vi "PowerDmm.vi"() -> ()   [LabVIEW 2015]
uses:
  <vilib>/RAFA Solutions/Rainbow Flat UI Controls Kit (Light)/Boolean/Radio Button.ctl
  <vilib>/RAFA Solutions/Rainbow Flat UI Controls Kit (Light)/Numeric/Numeric Indicator.ctl
  <vilib>/RAFA Solutions/Rainbow Flat UI Controls Kit (Light)/Numeric/Dial Simple.ctl
  <vilib>/RAFA Solutions/Rainbow Flat UI Controls Kit (Light)/Boolean/Slide Switch Round.ctl
  <vilib>/VirtualBench/_DMM Configure Measurement4.vi
  <vilib>/VirtualBench/_PS Configure Voltage Output0.vi
  <vilib>/VirtualBench/VirtualBench.lvlib
  <vilib>/RAFA Solutions/Rainbow Flat UI Controls Kit (Light)/Rainbow Light.lvlib
panel:
  in  "Auto Range Terminal":i32(ring) items=["Low", "High"]
  in  "Power Channel":tag="VB8012-3060439/ps/+6V"
  out "Analog Data":cluster{dbl[], dbl[]}(graph)
  in  "Voltage Level (V)":dbl(slide)=2.0 caption="Current Limit (no change)" scale=0.0..25.0
  in  "Current Limit (A)":dbl(slide)=0.1 caption="Current Limit (no change)" scale=0.0..1.0
  in  "milliseconds to wait":u32=30
  in  "deltaV":dbl=0.2 format="%#_13g"
  in  "Vlow":dbl format="%#_13g"
  in  "Vhigh":dbl=6.0 format="%#_13g"
  in  "Voltage Ramp":T1
  out "Actual Voltage Level":T2 scale=0.0..2.0
  out "Actual Current":T2 scale=0.0..2.0
  out "Calculated Resistance":T3
  out "DMM Reading":dbl(knob)=20.92102921572232 scale=0.0..25.0
  out "DMM Reading (Waveform)":dbl(graph)
  in  "Auto Range":T4=TRUE caption="Auto Range (no change)"
  in  "Function":i32(ring) caption="Function (no change)" items=["DC Volts", "AC Volts", "DC Current", "AC Current", "Resistance", "Diode"]
  in  "stop":bool
  in  "Enable Outputs":T4
  in  "Power Channel":tag="ps/+6V" caption="Channel"
  in  "Device Name":tag="VB8012-3060439"
  # "Power Supply Configuration"
  # "Power Supply Output"
  # "Digital Multimeter"
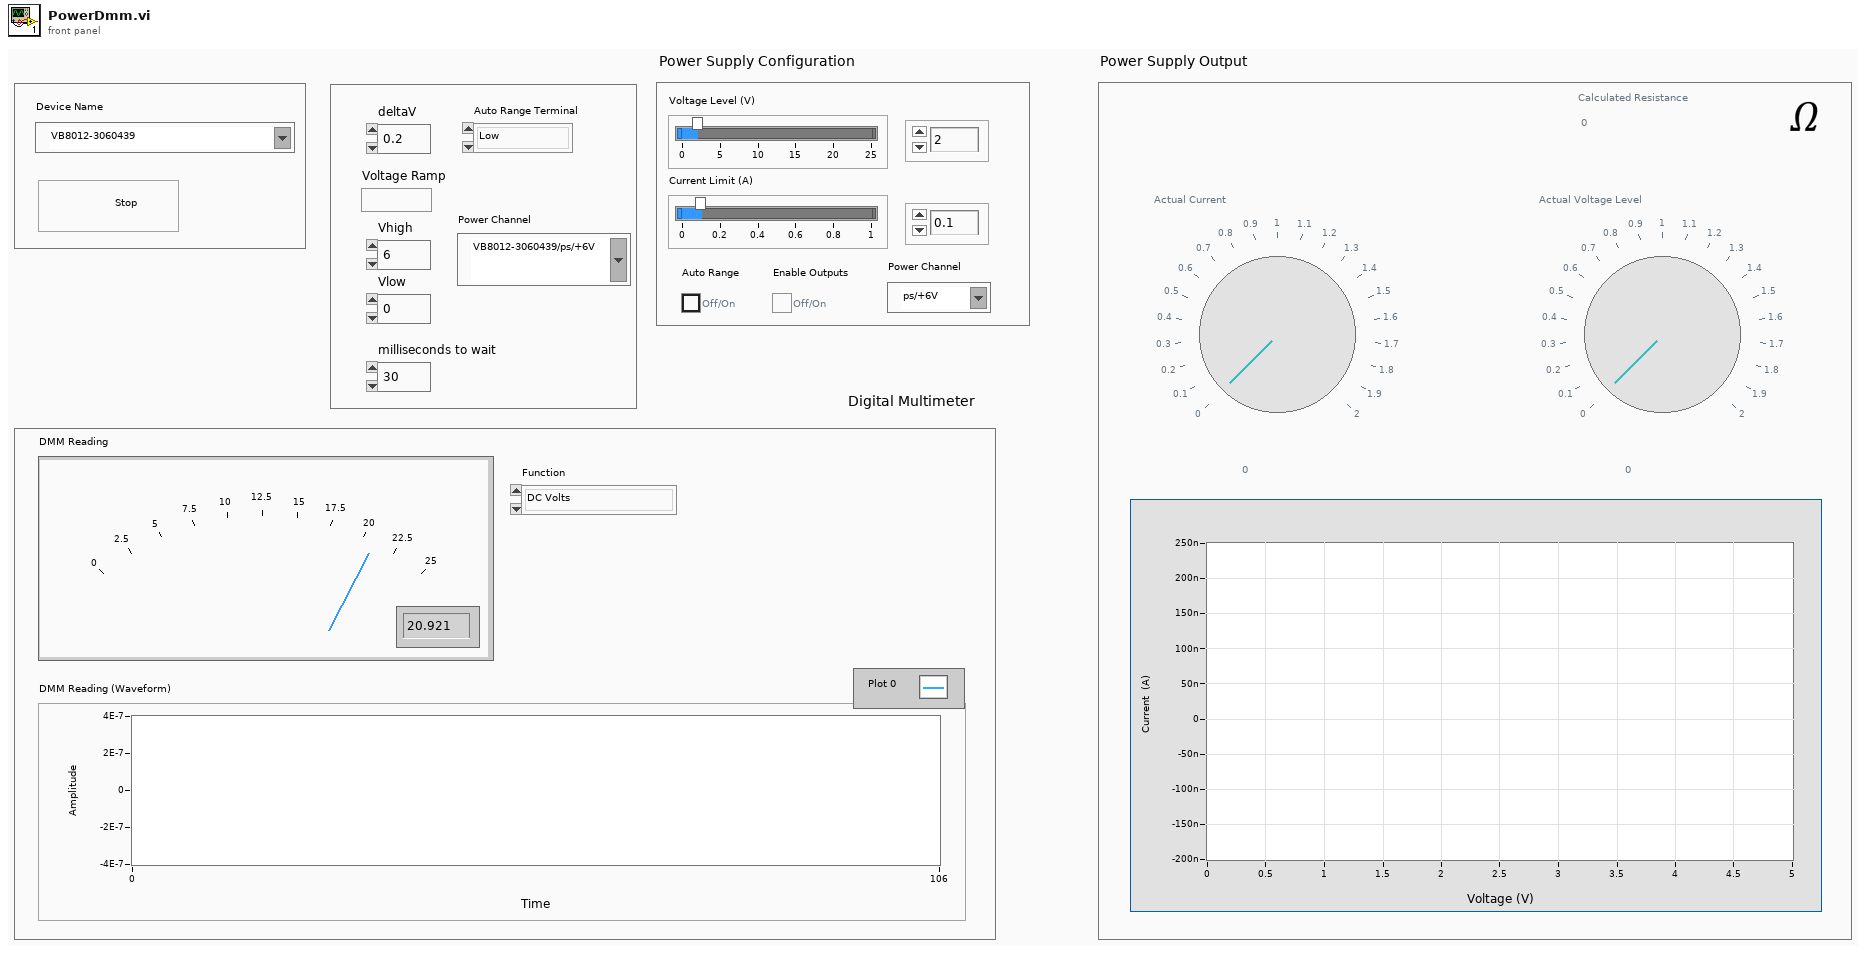
[diagram p1: front panel]
types:
  T1 = typedef "Rainbow Light.lvlib/Slide Switch Round.ctl" = bool
  T2 = typedef "Rainbow Light.lvlib/Dial Simple.ctl" = dbl
  T3 = typedef "Rainbow Light.lvlib/Numeric Indicator.ctl" = dbl
  T4 = typedef "Rainbow Light.lvlib/Radio Button.ctl" = bool
  T5 = cluster{"milliseconds to wait":u32, "deltaV":dbl, "Vhigh":dbl, "Vlow":dbl}
  T6 = cluster{"Instrument Handle Out":refnum<k21>, "Instrument Handle Out":refnum<k21>}
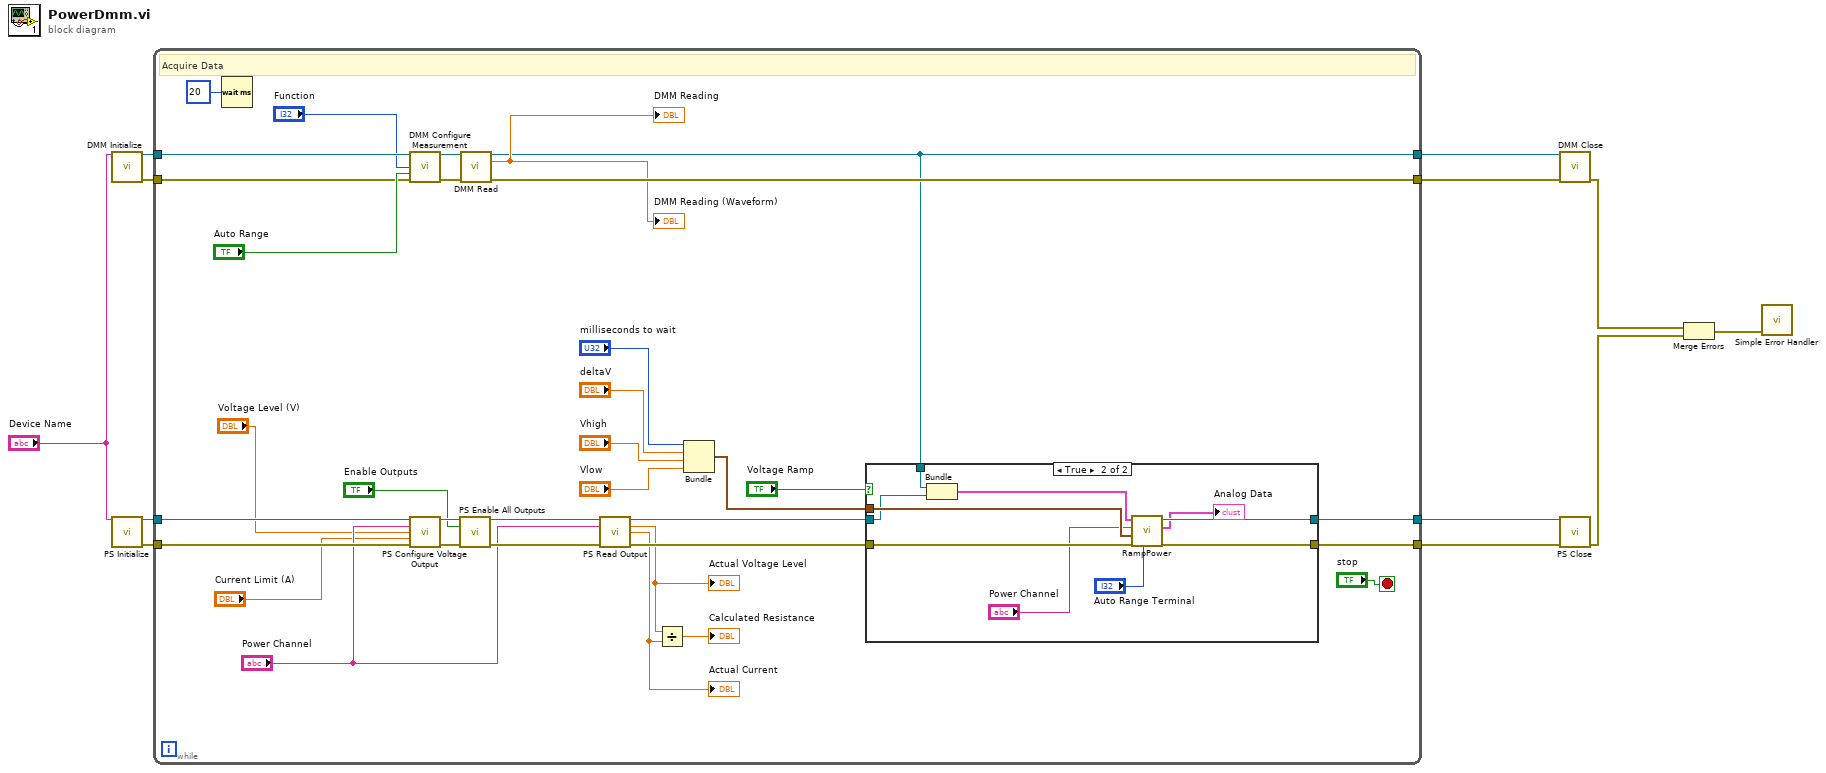
[diagram p0: block diagram]
diagram:
  n1 = call <vilib>:"DMM Initialize.vi"("Device Name"="Device Name") -> ("Instrument Handle Out"=w8:refnum<k21>, "Error Out"=w7:errorcluster)  [unwired: 13 in]
  n2 = call <vilib>:"PS Initialize.vi"("Device Name"="Device Name") -> ("Instrument Handle Out"=w12:refnum<k21>, "Error Out"=w11:errorcluster)  [unwired: 13 in]
  n3 = while {
    tunnel: w12 -> [w46]
    tunnel: w11 -> [w45]
    tunnel: [w27] -> w10
    tunnel: w8 -> [w39]
    tunnel: w7 -> [w35]
    tunnel: [w34] -> w6
    tunnel: [w26] -> w5
    tunnel: [w13] -> w4
    stop <- "stop" stop-if-true
    # "Acquire Data"
    n4 = Wait (ms)(milliseconds to wait=u32 20) -> ()  [unwired: 1 out]
    n5 = call-poly <vilib>:"DMM Configure Measurement.vi"("Instrument Handle In"=w39, "Function"="Function", "Auto Range"="Auto Range", "Error In"=w35) -> ("Instrument Handle Out"=w37:refnum<k21>, "Error Out"=w36:errorcluster)  [unwired: 10 in]
    n6 = call-poly <vilib>:"PS Configure Voltage Output.vi"("Instrument Handle In"=w46, "Channel"="Power Channel", "Voltage Level"="Voltage Level (V)", "Current Limit"="Current Limit (A)", "Error In"=w45) -> ("Instrument Handle Out"=w44:refnum<k21>, "Error Out"=w43:errorcluster)  [unwired: 9 in]
    n7 = call <vilib>:"PS Enable All Outputs.vi"("Instrument Handle In"=w44, "Enable Outputs"="Enable Outputs", "Error In"=w43) -> ("Instrument Handle Out"=w33:refnum<k21>, "Error Out"=w32:errorcluster)  [unwired: 11 in]
    n8 = call <vilib>:"DMM Read.vi"("Instrument Handle In"=w37, "Error In"=w36) -> ("Instrument Handle Out"=w13:refnum<k21>, "Measurement"=→"DMM Reading (Waveform)" →"DMM Reading":dbl, "Error Out"=w34:errorcluster)  [unwired: 11 in]
    n9 = call <vilib>:"PS Read Output.vi"("Instrument Handle In"=w33, "Channel"="Power Channel", "Error In"=w32) -> ("Instrument Handle Out"=w29:refnum<k21>, "Actual Voltage Level"=w17:dbl, "Actual Current Level"=w20:dbl, "Error Out"=w28:errorcluster)  [unwired: 8 in, 1 out]
    "Actual Current" <- w20
    "Actual Voltage Level" <- w17
    n10 = Divide(x=w17, y=w20) -> (x/y=→"Calculated Resistance":dbl)
    n11 = Bundle("milliseconds to wait"="milliseconds to wait", "deltaV"="deltaV", "Vhigh"="Vhigh", "Vlow"="Vlow") -> (w25:T5)  [unwired: 1 in]
    n12 = case shown="True" "Voltage Ramp" {
      tunnel: w29 -> [w48 w53]
      tunnel: w28 -> [w47 w58]
      tunnel: [w47 w57] -> w27
      tunnel: [w48 w56] -> w26
      tunnel: w25 -> [_ w55]
      tunnel: w13 -> [_ w52]
      frame False {
      }
      frame True {
        n13 = Bundle("Instrument Handle Out"=w52, "Instrument Handle Out"=w53) -> (w51:T6)  [unwired: 1 in]
        n14 = call "RampPower.vi"("Auto Range Terminal"="Auto Range Terminal", "Error In"=w58, "Cluster"=w55, "Power Channel"="Power Channel", "Instrument Handles"=w51) -> ("Error Out"=w57:errorcluster, "Voltage & Current"=→"Analog Data":cluster{dbl[], dbl[]}, "PWS Out"=w56:refnum<k21>)  [unwired: 4 in]
      }
    }
  }
  n15 = call <vilib>:"DMM Close.vi"("Instrument Handle In"=w4, "Error In"=w6) -> ("Error Out"=w3:errorcluster)  [unwired: 13 in]
  n16 = call <vilib>:"PS Close.vi"("Instrument Handle In"=w5, "Error In"=w10) -> ("Error Out"=w2:errorcluster)  [unwired: 13 in]
  n17 = Merge Errors(w3, w2) -> (w1:errorcluster)
  n18 = call <vilib>:"Simple Error Handler.vi"("error in (no error)"=w1) -> ()  [unwired: 4 in, 5 out]
